vi "ASCIIToBinary.vi"(8 "error in (no error)":errorcluster, 11 "VISA resource name":refnum<visa-resource-name>) -> (0 "error out":errorcluster, 3 "VISA resource name":refnum<visa-resource-name>)   [LabVIEW 2017, in "Sefram DAS220.lvlib"]
doc: "Switch to SCPI transaction to binary one."
uses:
  <instrlib>/Sefram DAS220/Sefram DAS220.lvlib
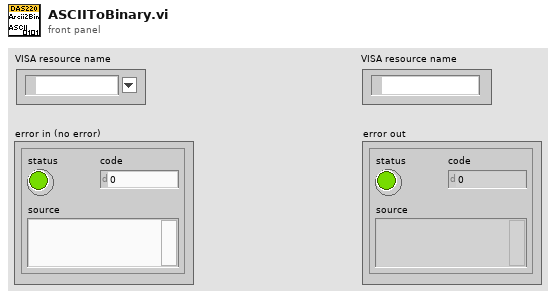
[diagram p1: front panel]
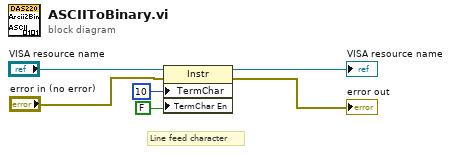
[diagram p0: block diagram]
diagram:
  # "Line feed character"
  n1 = property class="Instr"(reference="VISA resource name", error in="error in (no error)", "TermChar"=u8 10 ("Message Based Settings:Termination Character"), "TermChar En"=FALSE ("Message Based Settings:Termination Character Enable")) -> (reference out=→"VISA resource name":refnum<visa-resource-name>, error out=→"error out":errorcluster)
